vi "realtime (SubVI).vi"(6 "Min Value":dbl, 7 "Max Value":dbl, 9 "Start Collecting Real-Time Data":bool, 10 "Reset Real-Time Graph":bool, 11 "Refnum in":refnum<k21>) -> (1 "Current Voltage (mV)":dbl, 2 "Converted Temperature (C)":dbl, 3 "XY Graph":cluster{"X":dbl[], "Y":dbl[]}[](array[cluster]))   [LabVIEW 2020]
uses:
  <vilib>/ULx/Create Channel.llb/ULx Create Channel (AI-Voltage-Basic).vi
  <vilib>/ULx/Read.llb/ULx Read (Analog DBL 1Chan 1Samp).vi
  <vilib>/express/express arith-compare/Formula/XNode/ExpressFormulaBlockNode.xnode
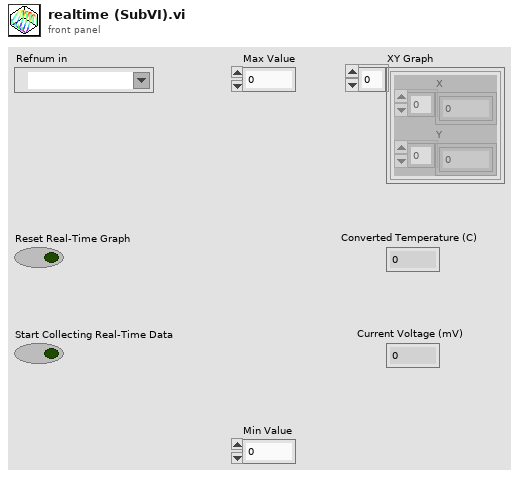
[diagram p1: front panel]
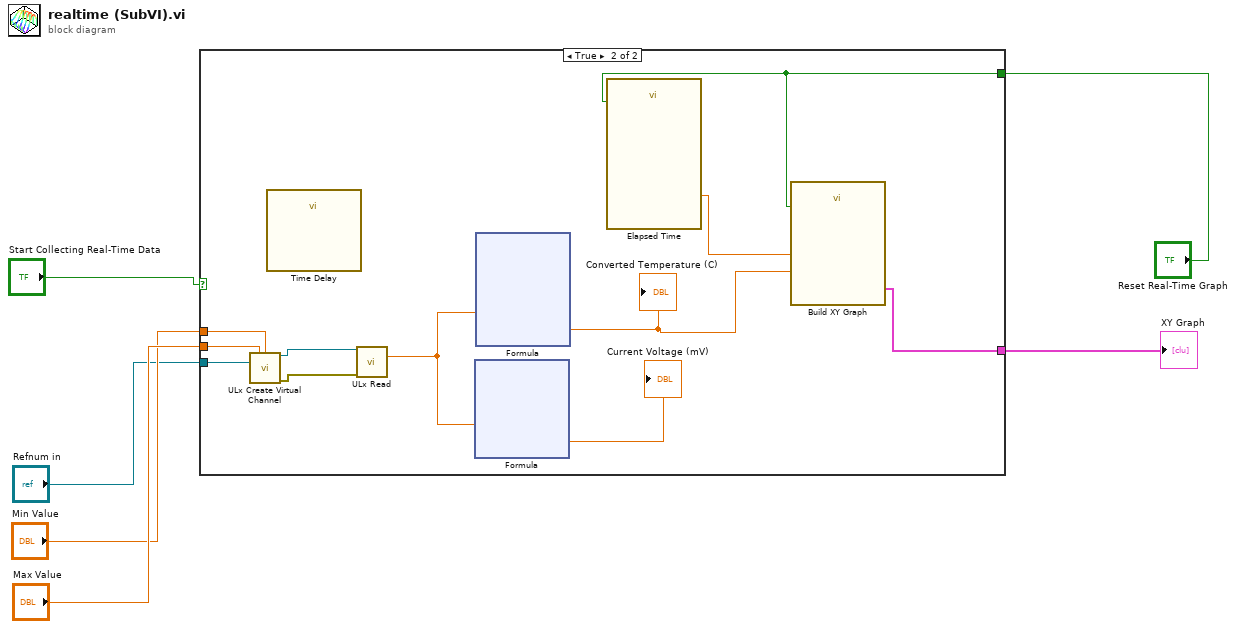
[diagram p0: block diagram]
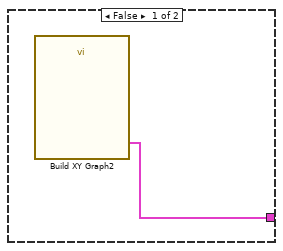
[diagram p2: hidden frame]
diagram:
  n1 = case shown="True" "Start Collecting Real-Time Data" {
    tunnel: "Refnum in" -> [_ w15]
    tunnel: "Min Value" -> [_ w14]
    tunnel: "Max Value" -> [_ w13]
    tunnel: [w7 w9] -> w5
    tunnel: "Reset Real-Time Graph" -> [_ w8]
    frame False {
      n2 = call "Build XY Graph2"() -> ("XY Graph"=w7:cluster{"X":dbl[], "Y":dbl[]}[])  [unwired: 10 in, 1 out]
    }
    frame True {
      n3 = call-poly <vilib>:"ULx Create Virtual Channel.vi"("maximum value"=w13, "minimum value"=w14, "physical channels"=w15) -> ("task out"=w12:refnum<k24>, "error out"=w11:errorcluster)  [unwired: 11 in]
      n4 = call "Time Delay"() -> ()  [unwired: 11 in, 1 out]
      n5 = call-poly <vilib>:"ULx Read.vi"("task in"=w12, "error in"=w11) -> ("data"=w18:dbl)  [unwired: 11 in, 2 out]
      n6 = xnode "Formula"("X1"=w18) -> ("Result"=→"Current Voltage (mV)":dbl)  [unwired: 1 in, 1 out]
      n7 = xnode "Formula"("X1"=w18) -> ("Result"=w16:dbl)  [unwired: 1 in, 1 out]
      "Converted Temperature (C)" <- w16
      n8 = call "Elapsed Time"("Reset"=w8) -> ("Elapsed Time (s)"=w10:dbl)  [unwired: 11 in, 7 out]
      n9 = call "Build XY Graph"("Reset"=w8, "Y Input"=w16, "X Input"=w10) -> ("XY Graph"=w9:cluster{"X":dbl[], "Y":dbl[]}[])  [unwired: 7 in, 1 out]
    }
  }
  "XY Graph" <- w5
